vi "clear_log.vi"(8 "error in":errorcluster, 11 "clear log?":bool) -> (0 "error out":errorcluster)   [LabVIEW 2013, in "Experiment.lvclass"]
uses:
  Experiment.lvclass
  Globals.vi
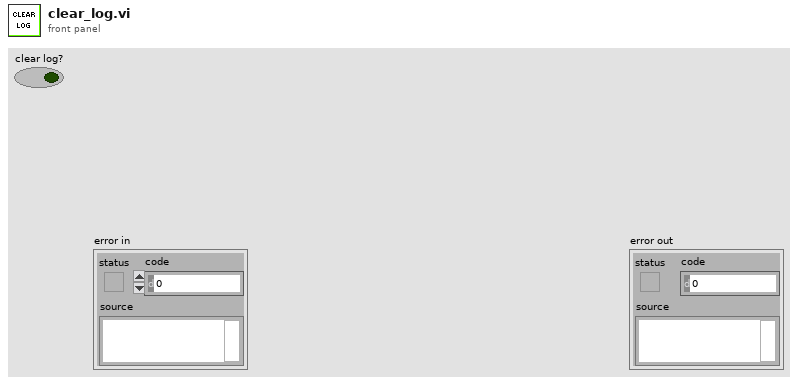
[diagram p1: front panel]
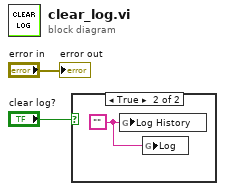
[diagram p0: block diagram]
diagram:
  n1 = case shown="True" "clear log?" {
    frame False {
    }
    frame True {
      w3 = ""
      n2 = global write "Globals.vi" "Log History"(w3) -> ()
      n3 = global write "Globals.vi" "Log"(w3) -> ()
    }
  }
  "error out" <- "error in"
